vi "ScanAction.vi"(8 "error in (no error)":errorcluster caption="entrée d'erreur (pas d'erreur)", 9 "IndicePoint":i32, 10 "Dir":bool, 11 "Tools In":refnum<class "Tools.lvclass"> caption="DNL_LabVIEW Object in") -> (0 "error out":errorcluster caption="sortie d'erreur", 2 "ScanParsOut":dbl[](array[numeric]), 3 "Tools Out":refnum<class "Tools.lvclass"> caption="DNL_LabVIEW Object out")   [LabVIEW 2019, in "Tools.lvclass"]
uses:
  Tools.lvclass
  C:/Programmes Labview/LabScanV1A/DevicesClass/BaseDevice/BaseDevice.lvclass
  Tools.lvclass/Tools.ctl
  <userlib>/GenProg/ReadbyWeakRefNum.vi
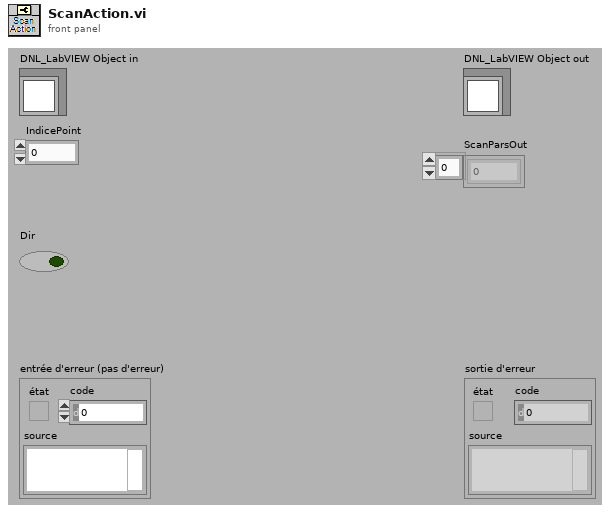
[diagram p1: front panel]
types:
  T1 = typedef "Tools.lvclass/Tools_Func.ctl" = enum16{"Courbe 1 (Arb)", "Courbe 2 (Arb)", "Courbe 3 (Arb)", "Courbe 123 (Arb,Arb,Arb)", "Scan Pos (Arb)", "Indice de Point (Points)", "AbsTime (ms)", "Minuteur (s)", "Panneaux Infos (Na)", "Délais (ms)", "RandwithDbind(Arb)", "RandomNum (Arb)", "Multisweep (Sw)", "ScanTime (s)"}
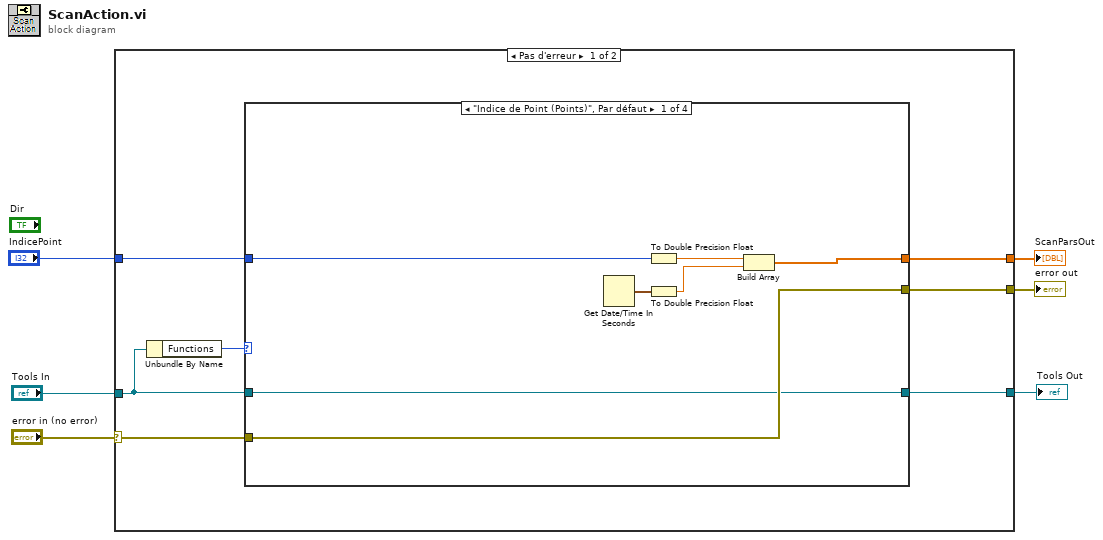
[diagram p0: block diagram]
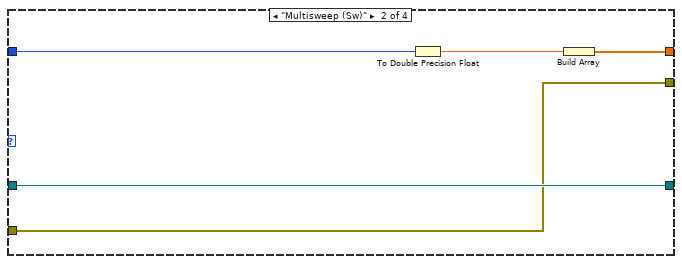
[diagram p2: hidden frame]
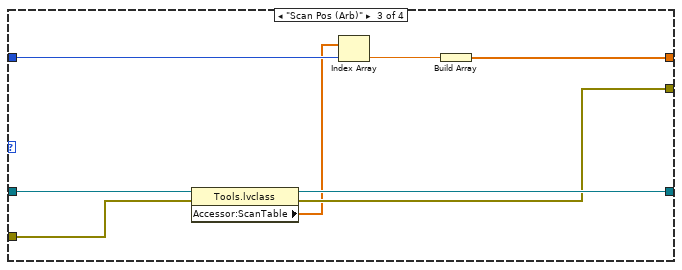
[diagram p3: hidden frame]
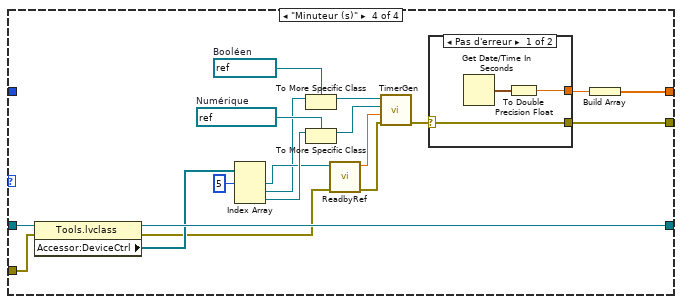
[diagram p4: hidden frame]
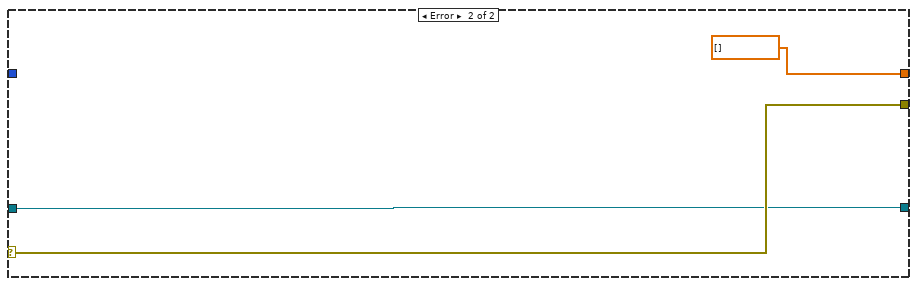
[diagram p6: hidden frame]
diagram:
  n1 = case shown="Pas d'erreur" "error in (no error)" {
    selector: "error in (no error)" -> [w10 w59]
    tunnel: "Tools In" -> [w11 w58]
    tunnel: [w9 dbl[] []] -> w1
    tunnel: [w8 w59] -> w4
    tunnel: [w7 w58] -> w3
    tunnel: "IndicePoint" -> [w12 _]
    frame No Error {
      n2 = Unbundle By Name(w11) -> ("Functions"=w13:T1)
      n3 = case shown="\"Indice de Point (Points)\", Par défaut" w13 {
        tunnel: [w19 w21 w26 w34] -> w9
        tunnel: w12 -> [w14 w25 w33 _]
        tunnel: [w15 w23 w30 w38] -> w7
        tunnel: w11 -> [w15 w23 w31 w39]
        tunnel: w10 -> [w20 w22 w29 w36]
        tunnel: [w20 w22 w28 w43] -> w8
        frame "Indice de Point (Points)", Default {
          n4 = Get Date/Time In Seconds() -> (seconds since 1Jan1904=w17:timestamp)
          n5 = To Double Precision Float(number=w14) -> (double precision float=w18:dbl)
          n6 = To Double Precision Float(number=w17) -> (double precision float=w16:dbl)
          n7 = Build Array(w18, w16) -> (w19:dbl[])
        }
        frame "Multisweep (Sw)" {
          n8 = To Double Precision Float(number=w25) -> (double precision float=w24:dbl)
          n9 = Build Array(w24) -> (w21:dbl[])
        }
        frame "Scan Pos (Arb)" {
          n10 = property class="Tools.lvclass"(reference=w31, error in=w29) -> (reference out=w30:refnum<class "Tools.lvclass">, error out=w28:errorcluster, "Accessor:ScanTable"=w27:dbl[])
          n11 = Index Array(array=w27, index=w33) -> (element=w32:dbl)
          n12 = Build Array(w32) -> (w26:dbl[])
        }
        frame "Minuteur (s)" {
          w49 = refnum<vi> refnum  # Numérique
          w51 = refnum<vi> refnum  # Booléen
          n13 = property class="Tools.lvclass"(reference=w39, error in=w36) -> (reference out=w38:refnum<class "Tools.lvclass">, error out=w35:errorcluster, "Accessor:DeviceCtrl"=w37:refnum<vi>[])
          n14 = Index Array(array=w37, index #1=5 ("indice")) -> (element #1=w41:refnum<vi>, element #2=w40:refnum<vi>, element #3=w48:refnum<vi>)  [unwired: 2 in]
          n15 = To More Specific Class(target class=w51, reference=w40) -> (specific class reference=w52:refnum<vi>)  [unwired: 1 in, 1 out]
          n16 = To More Specific Class(target class=w49, reference=w48) -> (specific class reference=w50:refnum<vi>)  [unwired: 1 in, 1 out]
          n17 = call-poly <userlib>:"ReadbyRef.vi"("error in"=w35, "Control Ref"=w41) -> ("error out"=w47:errorcluster, "Valeur"=w46:dbl)  [unwired: 8 in]
          n18 = call <userlib>:"TimerGen.vi"("error In"=w47, "Interval(s)"=w46, "TimeLeftRef"=w50, "UpdateRef"=w52) -> ("error out"=w44:errorcluster)  [unwired: 4 in, 3 out]
          n19 = case shown="Pas d'erreur" w44 {
            selector: w44 -> [w53 w56]
            tunnel: [w54 _] -> w45
            tunnel: [w53 w56] -> w43
            frame No Error {
              n20 = Get Date/Time In Seconds() -> (seconds since 1Jan1904=w55:timestamp)
              n21 = To Double Precision Float(number=w55) -> (double precision float=w54:dbl)
            }
            frame Error {
            }
          }
          n22 = Build Array(w45) -> (w34:dbl[])
        }
      }
    }
    frame Error {
    }
  }
  "error out" <- w4
  "Tools Out" <- w3
  "ScanParsOut" <- w1
